vi "Msg State Change.vi"(8 "error in":errorcluster, 10 "Transition State":refnum<class "Msg State Change.lvclass">, 11 "Msg State Change in":refnum<class "Msg State Change.lvclass">) -> (0 "error out":errorcluster, 3 "Msg State Change out":refnum<class "Msg State Change.lvclass">)   [LabVIEW 2021, in "Msg State Change.lvlib" / "Msg State Change.lvclass"]
uses:
  Msg State Change.lvclass
  C:/PPLs/Design-Patterns/State Pattern/State Pattern/State Pattern/State Pattern.lvclass
  State Pattern/State Pattern.lvclass
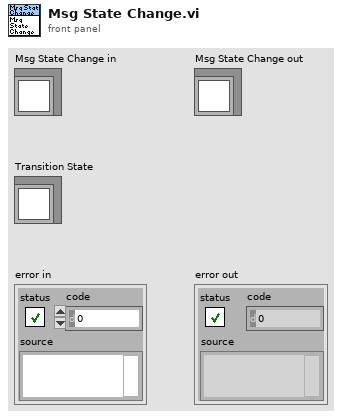
[diagram p1: front panel]
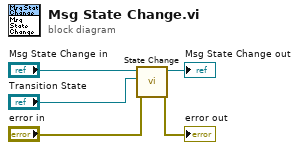
[diagram p0: block diagram]
diagram:
  n1 = call "State Change.vi"("error in"="error in", "Transition State"="Transition State", "Context in"="Msg State Change in") -> ("error out"=→"error out":errorcluster, "Context out"=→"Msg State Change out":refnum<class "Msg State Change.lvclass">)  [unwired: 7 in]
